vi "Initialize Sequence.vi"(6 "Listbox Ref In":refnum<vi>, 8 "error in (no error)":errorcluster, 10 "Seq Parameters":T1={"Test Name"="Unique Test Name", "Target"=enum."cRIO-9012", "Host IP Address"="0.0.0.0", "Target IP Address"="0.0.0.0", "Shared Variable Host"=enum."Target", "Shared Variable Writer"=enum."Target", "Variable Data Type"=enum."Double", "# of Variables per Library"=1, "Update Rate (Hz)"=1.0, "Read Rate (Hz)"=500.0, "Floor"=5000, "Ceiling"=500, "Delta"=500} {"# of Variables per Library" items=["50"=50, "100"=100, "150"=150, "200"=200, "250"=250, "300"=300, "350"=350, "400"=400, "450"=450, "500"=500]; "Delta" min=50 max=1000000 step=50; "Ceiling" min=50 max=1000000 step=50; "Floor" min=50 max=1000000 step=50}, 11 "SV B-M in":refnum<class "SV B-M (Host).lvclass">) -> (0 "error out":errorcluster, 3 "SV B-M out":refnum<class "SV B-M (Host).lvclass">, 5 "# of Tests":i32)   [LabVIEW 2015, in "SV B-M (Host).lvclass"]
doc: "Create a directory for this test, save this tests parameters as a configuration XML file, calculate the number of tests in the sequence and how many variables will be used in each test"
uses:
  SV B-M (Host).lvclass
  Type Defs/Sequence Parameters.ctl
  Type Defs/Target Type.ctl
  Type Defs/Variable Data Type.ctl
  SV B-M (Host).lvclass/SV B-M (Host).ctl
  Listbox - In Progress.vi
  Listbox - Complete.vi
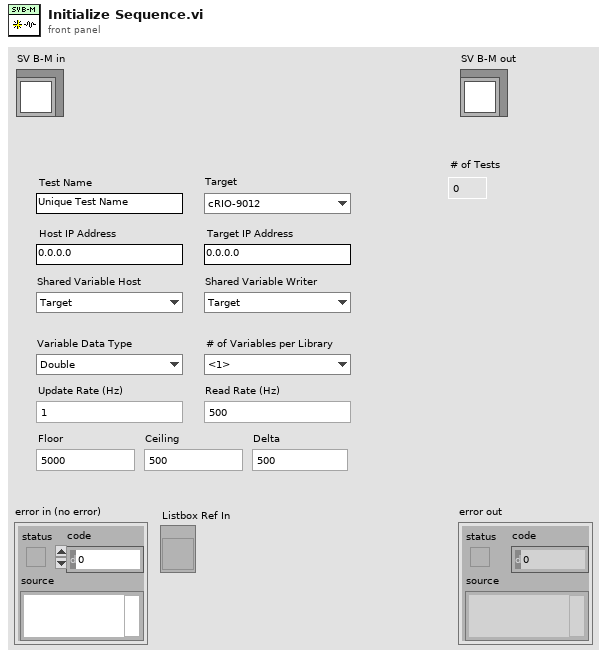
[diagram p1: front panel]
types:
  T1 = typedef "Sequence Parameters.ctl" = cluster{"Test Name":string, "Target":T2, "Host IP Address":string, "Target IP Address":string, "Shared Variable Host":enum16{"Target", "Host"}, "Shared Variable Writer":enum16{"Target", "Host"}, "Variable Data Type":T3, "# of Variables per Library":u16, "Update Rate (Hz)":dbl, "Read Rate (Hz)":dbl, "Floor":u32, "Ceiling":u32, "Delta":u32}
  T2 = typedef "Target Type.ctl" = enum16{"cRIO-9012", "cRIO-9014", "cRIO-9022", "cRIO-9023", "cRIO-9024", "cRIO-9025", "cRIO-9068", "cRIO-9073", "cRIO-9074", "cRIO-9075", "cRIO-9076", "cRIO-9081", "cRIO-9082", "myRIO-1900", "myRIO-1950", "PXI-8101", "PXI-8115", "PXI-8119", "PXI-8820", "PXIe-8100", "PXIe-8101", "PXIe-8133", "PXIe-8135", "PXIe-8820", "sbRIO-9605", "sbRIO-9606", "sbRIO-9623", "sbRIO-9626", "sbRIO-9633", "sbRIO-9636", "Unlisted (Linux-RT)", "Unlisted (PharLap)", "Unlisted (VxWorks)", "Windows Target"}
  T3 = typedef "Variable Data Type.ctl" = enum16{"U8", "U16", "U32", "U64", "I8", "I16", "I32", "I64", "Single", "Double", "Boolean", "String"}
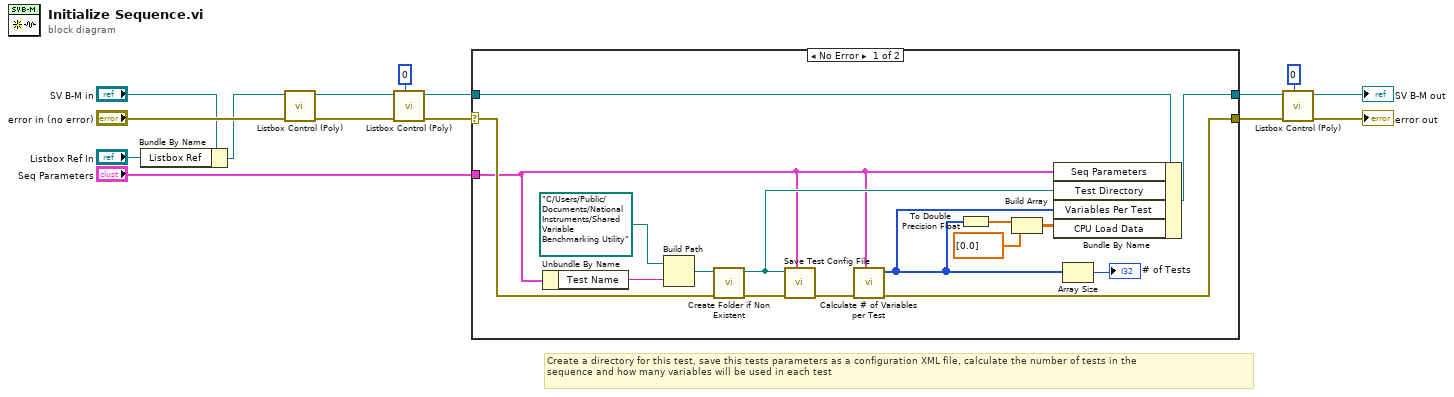
[diagram p0: block diagram]
diagram:
  # "Create a directory for this test, save this tests parameters as a configuration XML file, calculate the number of tests in the\nsequence and how many variables will be used in each test"
  n1 = Bundle By Name(cluster="SV B-M in", "Listbox Ref"="Listbox Ref In") -> (w1:refnum<class "SV B-M (Host).lvclass">)
  n2 = call-poly "Listbox Control (Poly).vi"("error in (no error)"="error in (no error)", "SV B-M In"=w1) -> ("error out"=w12:errorcluster, "SV B-M Out"=w13:refnum<class "SV B-M (Host).lvclass">)  [unwired: 8 in]
  n3 = call-poly "Listbox Control (Poly).vi"("Row to Update"=0, "error in (no error)"=w12, "SV B-M In"=w13) -> ("error out"=w5:errorcluster, "SV B-M Out"=w11:refnum<class "SV B-M (Host).lvclass">)  [unwired: 7 in]
  n4 = case shown="No Error" w5 {
    selector: w5 -> [w25 w32]
    tunnel: [w30 w33] -> w9
    tunnel: w11 -> [w31 w33]
    tunnel: "Seq Parameters" -> [w22 _]
    tunnel: [w20 w32] -> w4
    frame No Error {
      n5 = Unbundle By Name(w22) -> ("Test Name"=w28:string)
      n6 = Build Path(base path=path "C:/Users/Public/Documents/National Instruments/Shared Variable Benchmarking Utility", name or relative path=w28) -> (appended path=w27:path)
      n7 = call "Create Folder if Non Existent.vi"("error in (no error)"=w25, "Folder to Create"=w27) -> ("error out"=w26:errorcluster, "New Path Out"=w23:path)  [unwired: 8 in]
      n8 = call "Save Test Config File.vi"("Test Parameters"=w22, "error in (no error)"=w26, "Root Path"=w23) -> ("error out"=w24:errorcluster)  [unwired: 8 in]
      n9 = call "Calculate # of Variables per Test.vi"("Seq Parameters"=w22, "error in (no error)"=w24) -> ("error out"=w20:errorcluster, "# of Variables per Test"=w19:u32[])  [unwired: 8 in]
      n10 = To Double Precision Float(number=w19) -> (double precision float=w18:dbl[])
      n11 = Build Array(w18, dbl[] [0.0] ("element")) -> (w17:dbl[][])
      n12 = Bundle By Name(cluster=w31, "Seq Parameters"=w22, "Test Directory"=w23, "Variables Per Test"=w19, "CPU Load Data"=w17) -> (w30:refnum<class "SV B-M (Host).lvclass">)
      n13 = Array Size(array=w19) -> (size(s)=→"# of Tests":i32)
    }
    frame Error {
    }
  }
  n14 = call-poly "Listbox Control (Poly).vi"("Row to Update"=0, "error in (no error)"=w4, "SV B-M In"=w9) -> ("error out"=→"error out":errorcluster, "SV B-M Out"=→"SV B-M out":refnum<class "SV B-M (Host).lvclass">)  [unwired: 7 in]
